vi "CheckShotSuccess.vi"(6 "Vertical Edges":T2(array[cluster]) {"Point2 (Real-World)"."Y" format="%.2f"; "Point2 (Real-World)"."X" format="%.2f"; "Point1 (Real-World)"."Y" format="%.2f"; "Point1 (Real-World)"."X" format="%.2f"; "Point2 (Pixels)"."Y" format="%.2f"; "Point2 (Pixels)"."X" format="%.2f"; "Point1 (Pixels)"."Y" format="%.2f"; "Point1 (Pixels)"."X" format="%.2f"}, 8 "error in":errorcluster, 9 "File Path":path, 10 "CameraSettings":T4={"Brightness"=0, "Contrast"=0.0, "Threshold"=50.0}, 11 "Session In":T5) -> (0 "error out":errorcluster, 1 "Image":T1(plugin-control), 2 "Success?":bool, 3 "Session Out":T5)   [LabVIEW 2017]
uses:
  <vilib>/userdefined/High Color/IMAQdx.ctl
panel:
  out "Vertical Edges[0].Point1 (Pixels).X":sgl
  out "Circles[0].Position.X":sgl
  out "Puck":T3(array[cluster]) {"Position"."Y" format="%.2f"; "Position"."X" format="%.2f"}
  out "Number of Pucks Found":i32
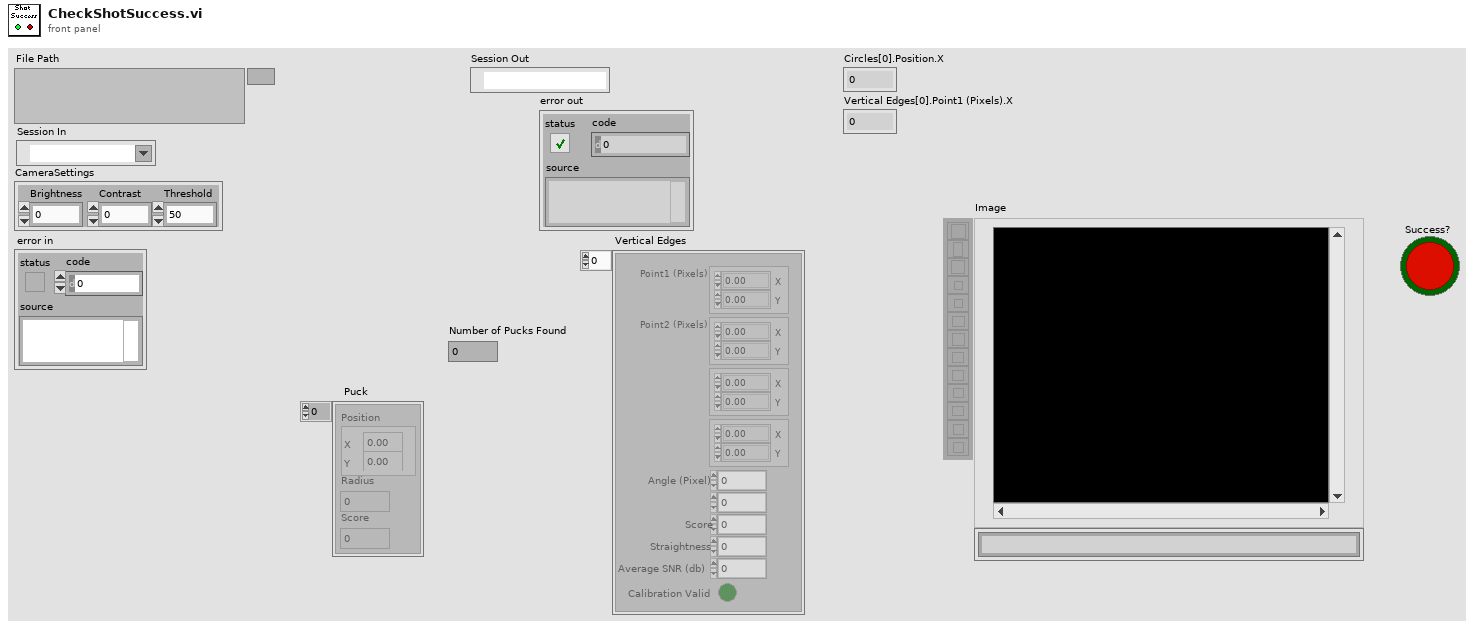
[diagram p1: front panel]
types:
  T1 = typedef "IMAQ Image.ctl" = refnum<image>
  T2 = cluster{"Point1 (Pixels)":cluster{"X":sgl, "Y":sgl}, "Point2 (Pixels)":cluster{"X":sgl, "Y":sgl}, "Point1 (Real-World)":cluster{"X":sgl, "Y":sgl}, "Point2 (Real-World)":cluster{"X":sgl, "Y":sgl}, "Angle (Pixel)":dbl, "Angle (Real-World)":dbl, "Score":dbl, "Straightness":dbl, "Average SNR (db)":dbl, "Calibration Valid":bool}[]
  T3 = cluster{"Position":cluster{"X":sgl, "Y":sgl}, "Radius":dbl, "Score":dbl}[]
  T4 = cluster{"Brightness":i64, "Contrast":dbl, "Threshold":sgl}
  T5 = typedef "IMAQdx.ctl" = refnum<k21>
  T6 = cluster{"Circles[0]":cluster{"Position":cluster{"X":sgl, "Y":sgl}, "Radius":dbl, "Score":dbl}, "Circles[1]":cluster{"Position":cluster{"X":sgl, "Y":sgl}, "Radius":dbl, "Score":dbl}, "Circles[2]":cluster{"Position":cluster{"X":sgl, "Y":sgl}, "Radius":dbl, "Score":dbl}, "Circles[3]":cluster{"Position":cluster{"X":sgl, "Y":sgl}, "Radius":dbl, "Score":dbl}, "Circles[4]":cluster{"Position":cluster{"X":sgl, "Y":sgl}, "Radius":dbl, "Score":dbl}, "Circles[5]":cluster{"Position":cluster{"X":sgl, "Y":sgl}, "Radius":dbl, "Score":dbl}, "Circles[6]":cluster{"Position":cluster{"X":sgl, "Y":sgl}, "Radius":dbl, "Score":dbl}, "Circles[7]":cluster{"Position":cluster{"X":sgl, "Y":sgl}, "Radius":dbl, "Score":dbl}, "Circles[8]":cluster{"Position":cluster{"X":sgl, "Y":sgl}, "Radius":dbl, "Score":dbl}}
  T7 = cluster{"Vertical Edges[0]":cluster{"Point1 (Pixels)":cluster{"X":sgl, "Y":sgl}, "Point2 (Pixels)":cluster{"X":sgl, "Y":sgl}, "Point1 (Real-World)":cluster{"X":sgl, "Y":sgl}, "Point2 (Real-World)":cluster{"X":sgl, "Y":sgl}, "Angle (Pixel)":dbl, "Angle (Real-World)":dbl, "Score":dbl, "Straightness":dbl, "Average SNR (db)":dbl, "Calibration Valid":bool}, "Vertical Edges[1]":cluster{"Point1 (Pixels)":cluster{"X":sgl, "Y":sgl}, "Point2 (Pixels)":cluster{"X":sgl, "Y":sgl}, "Point1 (Real-World)":cluster{"X":sgl, "Y":sgl}, "Point2 (Real-World)":cluster{"X":sgl, "Y":sgl}, "Angle (Pixel)":dbl, "Angle (Real-World)":dbl, "Score":dbl, "Straightness":dbl, "Average SNR (db)":dbl, "Calibration Valid":bool}, "Vertical Edges[2]":cluster{"Point1 (Pixels)":cluster{"X":sgl, "Y":sgl}, "Point2 (Pixels)":cluster{"X":sgl, "Y":sgl}, "Point1 (Real-World)":cluster{"X":sgl, "Y":sgl}, "Point2 (Real-World)":cluster{"X":sgl, "Y":sgl}, "Angle (Pixel)":dbl, "Angle (Real-World)":dbl, "Score":dbl, "Straightness":dbl, "Average SNR (db)":dbl, "Calibration Valid":bool}, "Vertical Edges[3]":cluster{"Point1 (Pixels)":cluster{"X":sgl, "Y":sgl}, "Point2 (Pixels)":cluster{"X":sgl, "Y":sgl}, "Point1 (Real-World)":cluster{"X":sgl, "Y":sgl}, "Point2 (Real-World)":cluster{"X":sgl, "Y":sgl}, "Angle (Pixel)":dbl, "Angle (Real-World)":dbl, "Score":dbl, "Straightness":dbl, "Average SNR (db)":dbl, "Calibration Valid":bool}, "Vertical Edges[4]":cluster{"Point1 (Pixels)":cluster{"X":sgl, "Y":sgl}, "Point2 (Pixels)":cluster{"X":sgl, "Y":sgl}, "Point1 (Real-World)":cluster{"X":sgl, "Y":sgl}, "Point2 (Real-World)":cluster{"X":sgl, "Y":sgl}, "Angle (Pixel)":dbl, "Angle (Real-World)":dbl, "Score":dbl, "Straightness":dbl, "Average SNR (db)":dbl, "Calibration Valid":bool}, "Vertical Edges[5]":cluster{"Point1 (Pixels)":cluster{"X":sgl, "Y":sgl}, "Point2 (Pixels)":cluster{"X":sgl, "Y":sgl}, "Point1 (Real-World)":cluster{"X":sgl, "Y":sgl}, "Point2 (Real-World)":cluster{"X":sgl, "Y":sgl}, "Angle (Pixel)":dbl, "Angle (Real-World)":dbl, "Score":dbl, "Straightness":dbl, "Average SNR (db)":dbl, "Calibration Valid":bool}, "Vertical Edges[6]":cluster{"Point1 (Pixels)":cluster{"X":sgl, "Y":sgl}, "Point2 (Pixels)":cluster{"X":sgl, "Y":sgl}, "Point1 (Real-World)":cluster{"X":sgl, "Y":sgl}, "Point2 (Real-World)":cluster{"X":sgl, "Y":sgl}, "Angle (Pixel)":dbl, "Angle (Real-World)":dbl, "Score":dbl, "Straightness":dbl, "Average SNR (db)":dbl, "Calibration Valid":bool}, "Vertical Edges[7]":cluster{"Point1 (Pixels)":cluster{"X":sgl, "Y":sgl}, "Point2 (Pixels)":cluster{"X":sgl, "Y":sgl}, "Point1 (Real-World)":cluster{"X":sgl, "Y":sgl}, "Point2 (Real-World)":cluster{"X":sgl, "Y":sgl}, "Angle (Pixel)":dbl, "Angle (Real-World)":dbl, "Score":dbl, "Straightness":dbl, "Average SNR (db)":dbl, "Calibration Valid":bool}, "Vertical Edges[8]":cluster{"Point1 (Pixels)":cluster{"X":sgl, "Y":sgl}, "Point2 (Pixels)":cluster{"X":sgl, "Y":sgl}, "Point1 (Real-World)":cluster{"X":sgl, "Y":sgl}, "Point2 (Real-World)":cluster{"X":sgl, "Y":sgl}, "Angle (Pixel)":dbl, "Angle (Real-World)":dbl, "Score":dbl, "Straightness":dbl, "Average SNR (db)":dbl, "Calibration Valid":bool}}
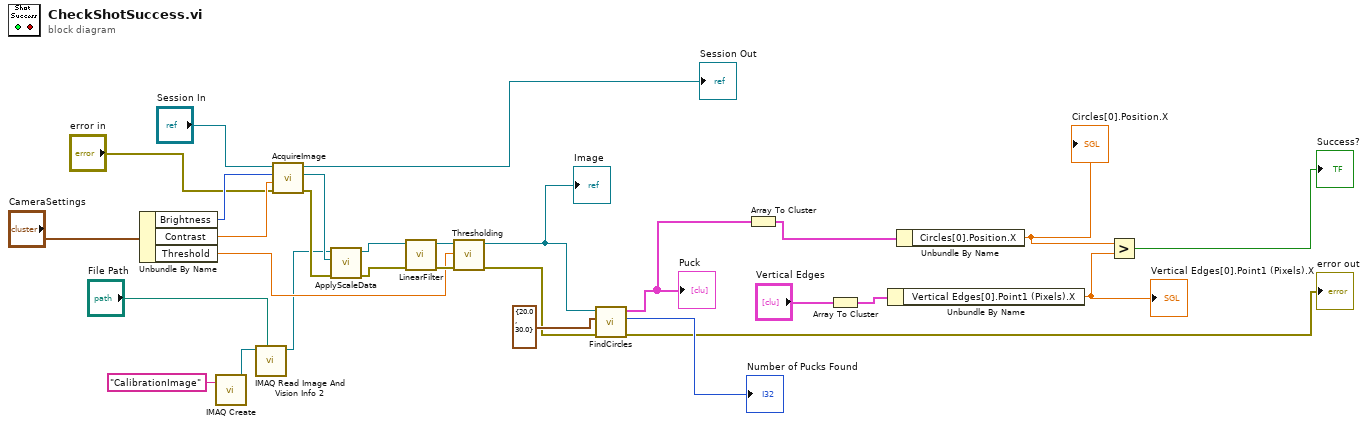
[diagram p0: block diagram]
diagram:
  n1 = Unbundle By Name("CameraSettings") -> ("Brightness"=w17:i64, "Contrast"=w16:dbl, "Threshold"=w14:sgl)
  n2 = call "IMAQ Create"("Image Name"="CalibrationImage") -> ("New Image"=w21:T1)  [unwired: 4 in, 1 out]
  n3 = call "IMAQ Read Image And Vision Info 2"("File Path"="File Path", "Image"=w21) -> ("Image Out"=w13:T1)  [unwired: 7 in, 2 out]
  n4 = call "AcquireImage.vi"("error in"="error in", "Contrast"=w16, "Brightness"=w17, "Session In"="Session In") -> ("error out"=w27:errorcluster, "Image"=w24:T1, "Session Out"=→"Session Out":T5)  [unwired: 4 in]
  n5 = call "ApplyScaleData.vi"("error in (no error)"=w27, "ImageIn"=w24, "CalibImage"=w13) -> ("error out"=w26:errorcluster, "Corrected Image"=w29:T1)  [unwired: 7 in]
  n6 = call "LinearFilter.vi"("error in (no error)"=w26, "Image Src"=w29) -> ("error out"=w25:errorcluster, "Image"=w28:T1)  [unwired: 8 in]
  n7 = call "Thresholding.vi"("error in (no error)"=w25, "Threshold Value"=w14, "Image Src"=w28) -> ("error out"=w3:errorcluster, "Image"=w1:T1)  [unwired: 7 in]
  "Image" <- w1
  n8 = call "FindCircles.vi"("error in (no error)"=w3, "Circle Descriptor"=cluster{"Max Radius":dbl, "Min Radius":dbl} {"Max Radius"=20.0, "Min Radius"=30.0}, "Image"=w1) -> ("error out"=→"error out":errorcluster, "Number of Matches Returned"=→"Number of Pucks Found":i32, "Circles"=w8:T3)  [unwired: 6 in]
  "Puck" <- w8
  n9 = Array To Cluster(array=w8) -> (cluster=w7:T6)
  n10 = Array To Cluster(array="Vertical Edges") -> (cluster=w9:T7)
  n11 = Unbundle By Name(w9) -> ("Vertical Edges[0].Point1 (Pixels).X"=w5:sgl)
  "Vertical Edges[0].Point1 (Pixels).X" <- w5
  n12 = Unbundle By Name(w7) -> ("Circles[0].Position.X"=w6:sgl)
  "Circles[0].Position.X" <- w6
  n13 = Greater?(x=w6, y=w5) -> (0:→"Success?":bool)
